vi "Format AK Command.vi"(8 "error in (no error)":errorcluster, 11 "String in":string) -> (0 "error out":errorcluster, 2 "Command":string, 3 "Command Code":string)   [LabVIEW 2013, in "Protocol Classes.lvlib"]
uses:
  Protocol Classes.lvlib
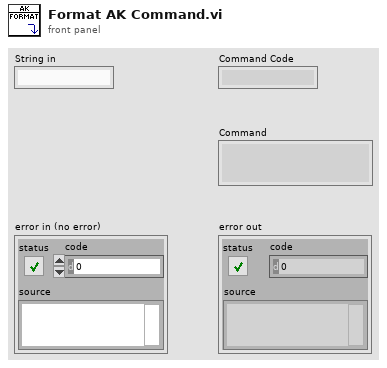
[diagram p1: front panel]
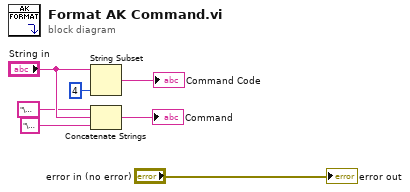
[diagram p0: block diagram]
diagram:
  n1 = String Subset(string="String in", length (rest)=4 ("length (rest)")) -> (substring=→"Command Code":string)  [unwired: 1 in]
  n2 = Concatenate Strings("\u0002 " ("string"), "String in", "\u0003" ("string")) -> (→"Command":string)
  "error out" <- "error in (no error)"
